vi "Validate Arguments.vi"(8 "error in (no error)":errorcluster, 11 "AddProjAction in":refnum<class "AddProjAction.lvclass">) -> (0 "error out":errorcluster, 2 "Problems":string[](array[string]), 3 "AddProjAction out":refnum<class "AddProjAction.lvclass">)   [LabVIEW 2020, in "AddProjAction.lvclass"]
uses:
  AddProjAction.lvclass
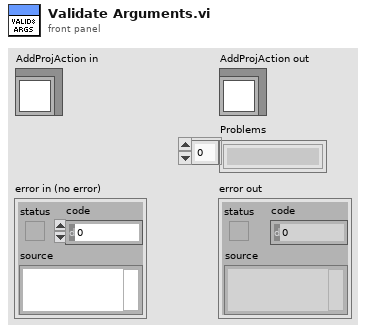
[diagram p1: front panel]
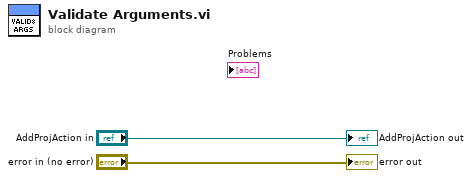
[diagram p0: block diagram]
diagram:
  "error out" <- "error in (no error)"
  "AddProjAction out" <- "AddProjAction in"
